vi "UnblockFile.vi"(0 "source path":path, 5 "error in (no error)":errorcluster) -> (19 "error out":errorcluster)   [LabVIEW 2012, in "G#Installer.lvlib"]
uses:
  G#Installer.lvlib
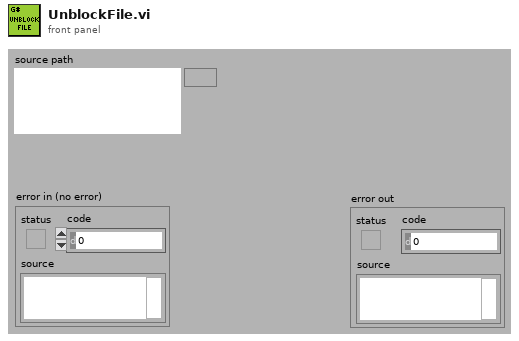
[diagram p1: front panel]
types:
  T1 = enum16{"open", "replace", "create", "open or create", "replace or create", "replace or create with confirmation"}
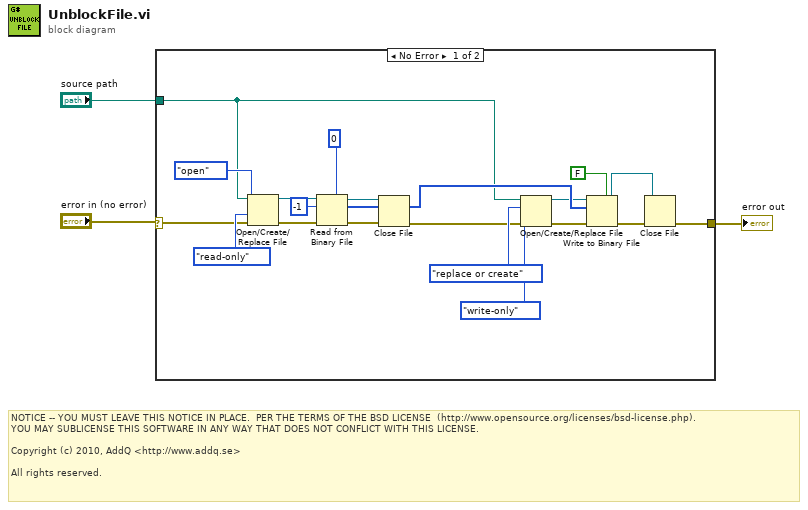
[diagram p0: block diagram]
diagram:
  # "NOTICE -- YOU MUST LEAVE THIS NOTICE IN PLACE.  PER THE TERMS OF THE BSD LICENSE  (http://www.opensource.org/licenses/bsd-license.php).\nYOU MAY SUBLICENSE THIS SOFTWARE IN ANY WAY THAT DOES NOT CONFLICT WITH THIS LICENSE.\n\nCopyright (c) 2010, AddQ <http://www.addq.se>\n\nAll rights reserved."
  n1 = case shown="No Error" "error in (no error)" {
    selector: "error in (no error)" -> [w4 w24]
    tunnel: "source path" -> [w10 _]
    tunnel: [w8 w24] -> w2
    frame No Error {
      n2 = Open/Create/Replace File(file path (use dialog)=w10, error in=w4, operation (0:open)=T1."open", access (0:read/write)=enum16{"read/write", "read-only", "write-only"}."read-only") -> (refnum out=w22:refnum<file>, error out=w21:errorcluster)  [unwired: 2 in, 1 out]
      n3 = Read from Binary File(5:u8 0, 8:w21, 10:-1 ("count (1)"), 11:w22) -> (0:w12:errorcluster, 2:w18:u8[], 3:w11:refnum<file>)  [unwired: 2 in, 1 out]
      n4 = Close File(refnum=w11, error in=w12) -> (error out=w5:errorcluster)  [unwired: 1 out]
      n5 = Open/Create/Replace File(file path (use dialog)=w10, error in=w5, operation (0:open)=T1."replace or create", access (0:read/write)=enum16{"read/write", "read-only", "write-only"}."write-only") -> (refnum out=w17:refnum<file>, error out=w19:errorcluster)  [unwired: 2 in, 1 out]
      n6 = Write to Binary File(file (use dialog)=w17, data=w18, error in=w19, 5:FALSE ("prepend array or string size? (T)")) -> (refnum out=w16:refnum<file>, error out=w9:errorcluster)  [unwired: 2 in, 1 out]
      n7 = Close File(refnum=w16, error in=w9) -> (error out=w8:errorcluster)  [unwired: 1 out]
    }
    frame Error {
    }
  }
  "error out" <- w2
